vi "Tone.vi"(0 "Arduino Resource":T1={"VISA resource"="", "Board Type"=enum."Arduino Uno", "Connection Type"=enum."USB / Serial", "Bytes Per Packet (15)"=15}, 5 "Tone DO Pin":u8=8, 7 "Frequency (0 Hz)":u16 step=100, 9 "Duration (1 ms)":u32=50, 11 "error in":errorcluster) -> (4 "Arduino Resource":T1={"VISA resource"="", "Board Type"=enum."Arduino Uno", "Connection Type"=enum."USB / Serial", "Bytes Per Packet (15)"=15}, 15 "error out":errorcluster)   [LabVIEW 2011, in "LabVIEW Interface for Arduino.lvlib"]
doc: "Generates a square wave with the specified frequency and 50% duty cycle. Use this VI with frequency equal to 0 to stop the signal generation on the specified pin. This command can only be used on one pin at a time and signal generation must be stopped on one pin before it can be started on another."
uses:
  <vilib>/LabVIEW Interface for Arduino/LabVIEW Interface for Arduino.lvlib
  <vilib>/LabVIEW Interface for Arduino/Private/Type Defs/Arduino Resource.ctl
  <vilib>/LabVIEW Interface for Arduino/Private/Type Defs/Board Type.ctl
  <vilib>/LabVIEW Interface for Arduino/Private/Type Defs/Command.ctl
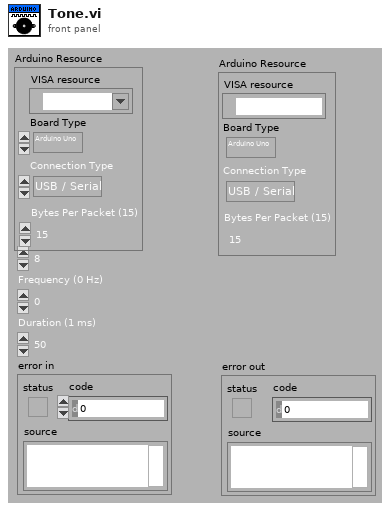
[diagram p1: front panel]
types:
  T1 = typedef "LabVIEW Interface for Arduino.lvlib/Arduino Resource.ctl" = cluster{"VISA resource":refnum<visa-resource-name>, "Board Type":T2, "Connection Type":enum8{"USB / Serial"}, "Bytes Per Packet (15)":u8}
  T2 = typedef "LabVIEW Interface for Arduino.lvlib/Board Type.ctl" = enum16{"Arduino Uno", "Dimuelanove w/Atmega 328", "Mega 2560", "Chipkit Uno32", "Chipkit Max32"}
  T3 = typedef "LabVIEW Interface for Arduino.lvlib/Command.ctl" = enum8{"setArduinoMode", "flushSerial", "setPinMode", "digitalWritePin", "digitalWritePort", "tone", "digitalReadPin", "digitalReadPort", "analogReadPin", "analogReadPort", "pwmWritePin", "pwmWritePort", "sevenSegment_Configure", "sevenSegment_Write", "I2C Init", "I2C Write", "I2C Read", "SPI Init", "SPI Set Bit Order", "SPI Set Clock Divider", "SPI Set Data Mode", "SPI Send / Receive", "SPI Close", "Servo Set Num Servos", "Servo Config Servo", "Servo Write Angle", "Servo Read Angle", "Servo Write Pulse Width", "Servo Read Pulse Width", "Servo Detach", "LCD Init", "LCD Set Size", "LCD Set Cursor Mode", "LCD Clear", "LCD Set Cursor Position", "LCD Print", "LCD Display Power", "LCD Scroll Display", "LCD Autoscroll", "LCD Print Direction", "LCD Create Custom Char", "LCD Print Custom Char", "contAcqOn", "contAcqOff", "getFirmwareVersion", "FiniteSampleStart"}
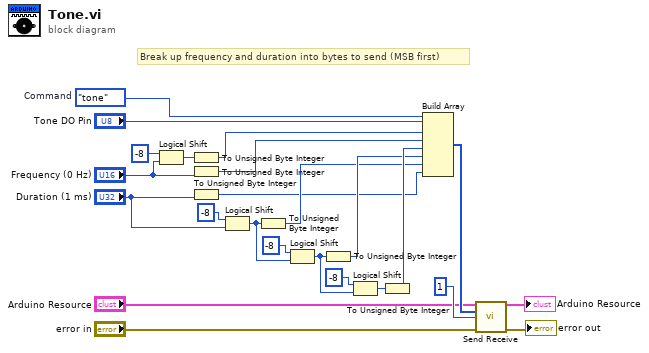
[diagram p0: block diagram]
diagram:
  w1 = Command."tone"  # Command
  # "Break up frequency and duration into bytes to send (MSB first)"
  n1 = Logical Shift(y=i8 -8, x="Frequency (0 Hz)") -> (x << y=w9:u16)
  n2 = To Unsigned Byte Integer(number=w9) -> (unsigned 8bit integer=w10:u8)
  n3 = To Unsigned Byte Integer(number="Frequency (0 Hz)") -> (unsigned 8bit integer=w7:u8)
  n4 = To Unsigned Byte Integer(number="Duration (1 ms)") -> (unsigned 8bit integer=w12:u8)
  n5 = Logical Shift(y=i8 -8, x="Duration (1 ms)") -> (x << y=w17:u32)
  n6 = To Unsigned Byte Integer(number=w17) -> (unsigned 8bit integer=w13:u8)
  n7 = Logical Shift(y=i8 -8, x=w17) -> (x << y=w18:u32)
  n8 = To Unsigned Byte Integer(number=w18) -> (unsigned 8bit integer=w19:u8)
  n9 = Logical Shift(y=i8 -8, x=w18) -> (x << y=w16:u32)
  n10 = To Unsigned Byte Integer(number=w16) -> (unsigned 8bit integer=w20:u8)
  n11 = Build Array(w1, "Tone DO Pin", w10, w7, w20, w19, w13, w12) -> (w21:u8[])
  n12 = call <vilib>:"Send Receive.vi"("Arduino Resource"="Arduino Resource", "Data"=w21, "Bytes To Read (0)"=u8 1, "error in"="error in") -> ("Arduino Resource"=→"Arduino Resource":T1, "error out"=→"error out":errorcluster)  [unwired: 9 in, 1 out]
